vi "Audio Playback Example (L+R).vi"() -> ()   [LabVIEW 2020]
doc: "Simple example of audio device playback of a file decoded with G-Audio."
uses:
  <vilib>/Dataflow_G/G-Audio/Controls/Audio Device Config.ctl
  <vilib>/Dataflow_G/G-Audio/Controls/Audio Device Format.ctl
  <vilib>/Dataflow_G/G-Audio/Controls/Audio Device Info.ctl
  <vilib>/Dataflow_G/G-Audio/Controls/Audio Device Type.ctl
  0e12f40e-f14c-4290-a5ea-138866c441b1.vi
  d7e0c978-9125-405d-aeed-362ffa71d3ba.vi
  <vilib>/Dataflow_G/G-Audio/Private/Get Basic Audio File Info.vi
  <vilib>/Dataflow_G/G-Audio/Private/Result To Error.vi
  0e12f40e-f14c-4290-a5ea-138866c441b1.vi/83e036c8-5b8f-4422-8bad-29d1a5d88806.vi
  <vilib>/Dataflow_G/G-Audio/Private/Audio File Refnum To Value.vi
  0e12f40e-f14c-4290-a5ea-138866c441b1.vi/d9ec978b-e613-4283-b939-906631cbae9f.vi
  <vilib>/Dataflow_G/G-Audio/Private/Audio Device Refnum To Value.vi
  d7e0c978-9125-405d-aeed-362ffa71d3ba.vi/8d74a8f2-5c3d-4df2-821e-21dd244a6609.vi
  d7e0c978-9125-405d-aeed-362ffa71d3ba.vi/7061ddd9-0afb-4971-a4a2-245ae16bf67f.vi
  0e12f40e-f14c-4290-a5ea-138866c441b1.vi/d9ec978b-e613-4283-b939-906631cbae9f.vi/a7c7f5a1-14d3-4370-a942-7aad9956b608.vi
  d7e0c978-9125-405d-aeed-362ffa71d3ba.vi/8d74a8f2-5c3d-4df2-821e-21dd244a6609.vi/a7c7f5a1-14d3-4370-a942-7aad9956b608.vi
  d7e0c978-9125-405d-aeed-362ffa71d3ba.vi/7061ddd9-0afb-4971-a4a2-245ae16bf67f.vi/54365fae-8b7b-405c-8b4a-440083926c8e.vi
  <vilib>/Utility/Data Type/Get Numeric Information.vi
  <vilib>/Utility/error.llb/Error Cluster From Error Code.vi
  <vilib>/Dataflow_G/G-Audio/Audio Files/Polymorphic VIs/Open Audio File Read (Path).vi
  <vilib>/Dataflow_G/G-Audio/G-Audio.lvlib
panel:
  in  "Right":sgl(slide)=1.0 scale=0.0..1.0
  in  "Left":sgl(slide)=1.0 scale=0.0..1.0
  out "Waveform":waveform(sgl)[](graph)
  out "error out":errorcluster
  in  "Stop":bool
  # "Instructions:\n1. Run the VI.\n2. Select an audio file to play.\n3. The VI will stop when the file has finished playing, or when the Stop button is pressed."
  # "G"
  # "-Audio"
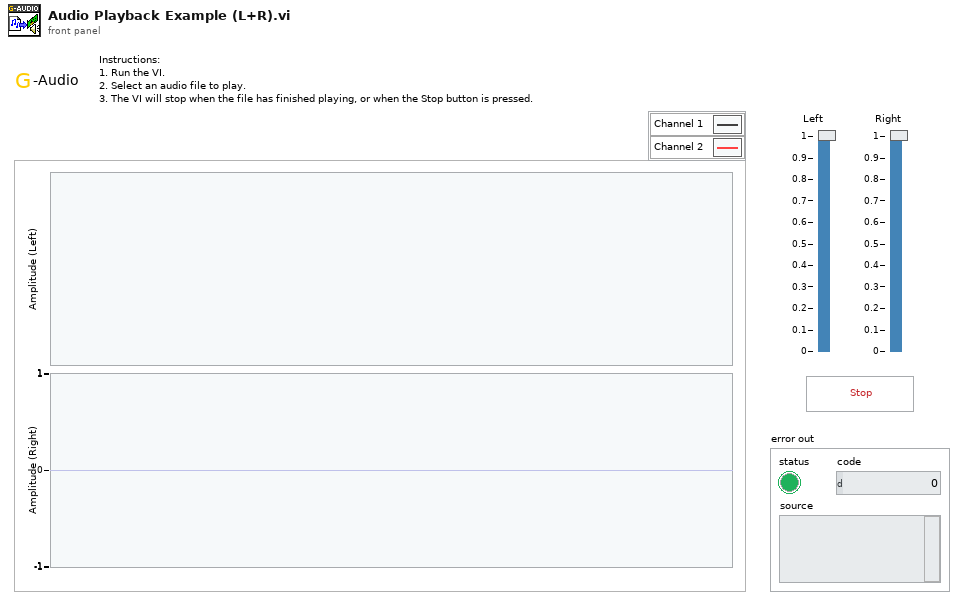
[diagram p1: front panel]
types:
  T1 = typedef "G-Audio.lvlib/Audio Device Info.ctl" = cluster{"Name":string, "ID":u8[], "Device Type":T2}
  T2 = typedef "G-Audio.lvlib/Audio Device Type.ctl" = enum16{"(None)", "Playback", "Capture", "Duplex", "Loopback"}
  T3 = typedef "G-Audio.lvlib/Audio Device Config.ctl" = cluster{"Sample Rate (Hz)":u32, "Channels":u32, "Format":T4, "Exclusive Mode":bool}
  T4 = typedef "G-Audio.lvlib/Audio Device Format.ctl" = enum16{"Native", "U8", "I16", "I32", "SGL"}
  T5 = typedef "G-Audio.lvlib/Audio File Refnum.ctl" = refnum<file>
  T6 = typedef "G-Audio.lvlib/Audio Device Refnum.ctl" = refnum<file>
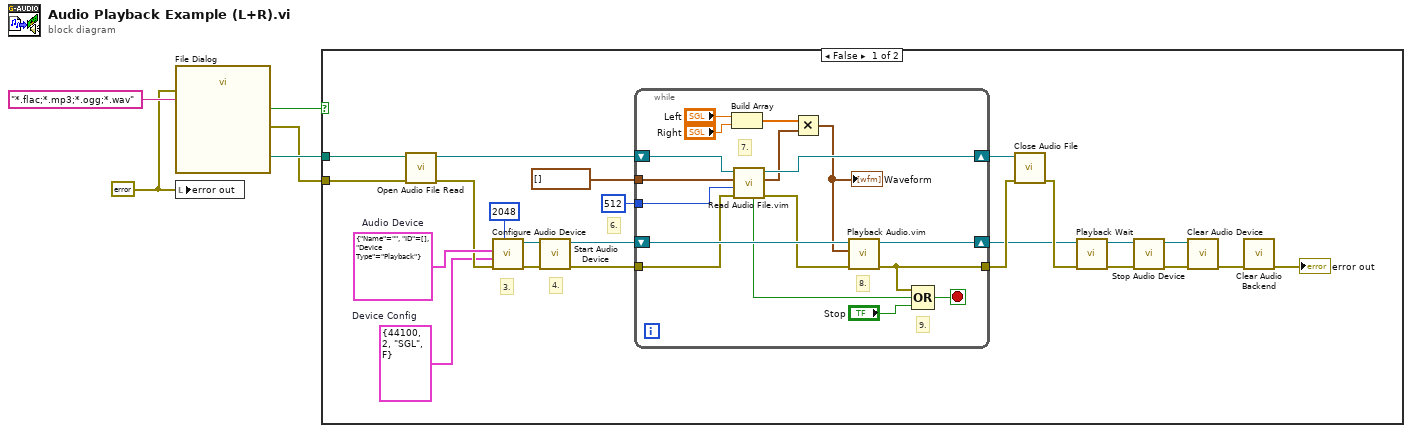
[diagram p0: block diagram]
diagram:
  w1 = errorcluster {"status"=FALSE, "code"=0, "source"=""} ("error out")
  n1 = call "File Dialog"("error in"=w1, "pattern (all files)"="*.flac;*.mp3;*.ogg;*.wav") -> ("selected path"=w4:path, "cancelled"=w3:bool, "error out"=w2:errorcluster)  [unwired: 10 in, 1 out]
  n2 = local write "error out"(w1) -> ()
  n3 = case shown="False" w3 {
    tunnel: w4 -> [w7 _]
    tunnel: w2 -> [w28 _]
    frame False {
      w12 = T1 {"Name"="", "ID"=[], "Device Type"=enum."Playback"}  # Audio Device
      w10 = T3 {"Sample Rate (Hz)"=44100, "Channels"=2, "Format"=enum."SGL", "Exclusive Mode"=FALSE}  # Device Config
      # "6."
      # "4."
      # "3."
      n4 = call-poly <vilib>:"Open Audio File Read.vi"("error in (no error)"=w28, "Path"=w7) -> ("error out"=w11:errorcluster, "Audio File Refnum"=w19:T5)  [unwired: 8 in]
      n5 = call <vilib>:"Configure Audio Device.vi"("Buffer Size (4096)"=2048 ("number of samples/ch"), "error in (no error)"=w11, "Device Config"=w10, "Audio Device"=w12) -> ("error out"=w18:errorcluster, "Audio Device Refnum"=w17:T6)  [unwired: 6 in]
      n6 = call <vilib>:"Start Audio Device.vi"("error in (no error)"=w18, "Audio Device Refnum In"=w17) -> ("error out"=w21:errorcluster, "Audio Device Refnum Out"=w22:T6)  [unwired: 8 in]
      n7 = while {
        shift-right: [w43] -> w27
        shift-left: w19 -> [w45]
        shift-right: [w42] -> w14
        shift-left: w22 -> [w44]
        tunnel: w21 -> [w41]
        tunnel: [w36] -> w25
        tunnel: u64 512 ("number of samples/ch") -> [w35]
        tunnel: waveform(sgl)[] [] -> [w32]
        stop <- w38 stop-if-true
        # "9."
        # "8."
        # "7."
        n8 = Build Array("Left", "Right") -> (w31:sgl[])
        n9 = call "Read Audio File.vim"("error in (no error)"=w41, "Frames To Read"=w35, "Data Format"=w32, "Audio File Refnum In"=w45) -> ("error out"=w40:errorcluster, "Audio Data"=w30:waveform(sgl)[], "Audio File Refnum Out"=w43:T5, "End of File?"=w39:bool)  [unwired: 3 in, 1 out]
        n10 = Multiply(x=w31, y=w30) -> (x*y=w29:waveform(sgl)[])
        "Waveform" <- w29
        n11 = call "Playback Audio.vim"("error in (no error)"=w40, "Audio Data"=w29, "Audio Device Refnum In"=w44) -> ("error out"=w36:errorcluster, "Audio Device Refnum Out"=w42:T6)  [unwired: 7 in]
        n12 = Compound Arithmetic op=OR(w36, w39, "Stop") -> (w38:bool)
      }
      n13 = call <vilib>:"Close Audio File.vi"("error in (no error)"=w25, "Audio File Refnum In"=w27) -> ("error out"=w24:errorcluster)  [unwired: 9 in]
      n14 = call <vilib>:"Playback Wait.vi"("error in (no error)"=w24, "Audio Device Refnum In"=w14) -> ("error out"=w15:errorcluster, "Audio Device Refnum Out"=w13:T6)  [unwired: 8 in]
      n15 = call <vilib>:"Stop Audio Device.vi"("error in (no error)"=w15, "Audio Device Refnum In"=w13) -> ("error out"=w23:errorcluster, "Audio Device Refnum Out"=w26:T6)  [unwired: 8 in]
      n16 = call <vilib>:"Clear Audio Device.vi"("error in (no error)"=w23, "Audio Device Refnum In"=w26) -> ("error out"=w20:errorcluster)  [unwired: 9 in]
      n17 = call <vilib>:"Clear Audio Backend.vi"("error in (no error)"=w20) -> ("error out"=→"error out":errorcluster)  [unwired: 10 in]
    }
    frame True {
    }
  }
